vi "getFTData.vi"(4 "Transformed Calibration Matrix":dbl[][](array[numeric]), 5 "error in":errorcluster, 6 "Bias Vector":dbl[](array[numeric])=[0.0, 0.0, 0.0, 0.0, 0.0, 0.0], 7 "Timing parameters":T1={"Sample Rate"=1000.0, "Samples to Read"=100}, 8 "task in":refnum<k21>) -> (0 "error out":errorcluster, 1 "Voltages":dbl[][](array[numeric]), 2 "F/T":dbl[][](array[numeric]) format="%0.4f", 3 "task out 2":refnum<k21>)   [LabVIEW 2012]
uses:
  <vilib>/DAQmx/read.llb/DAQmx Read (Analog 2D DBL NChan NSamp).vi
  <vilib>/DAQmx/miscellaneous.llb/DAQmx Fill In Error Info.vi
  <vilib>/Analysis/baseanly.llb/A x Vector.vi
  <vilib>/Analysis/NI_AALBase.lvlib
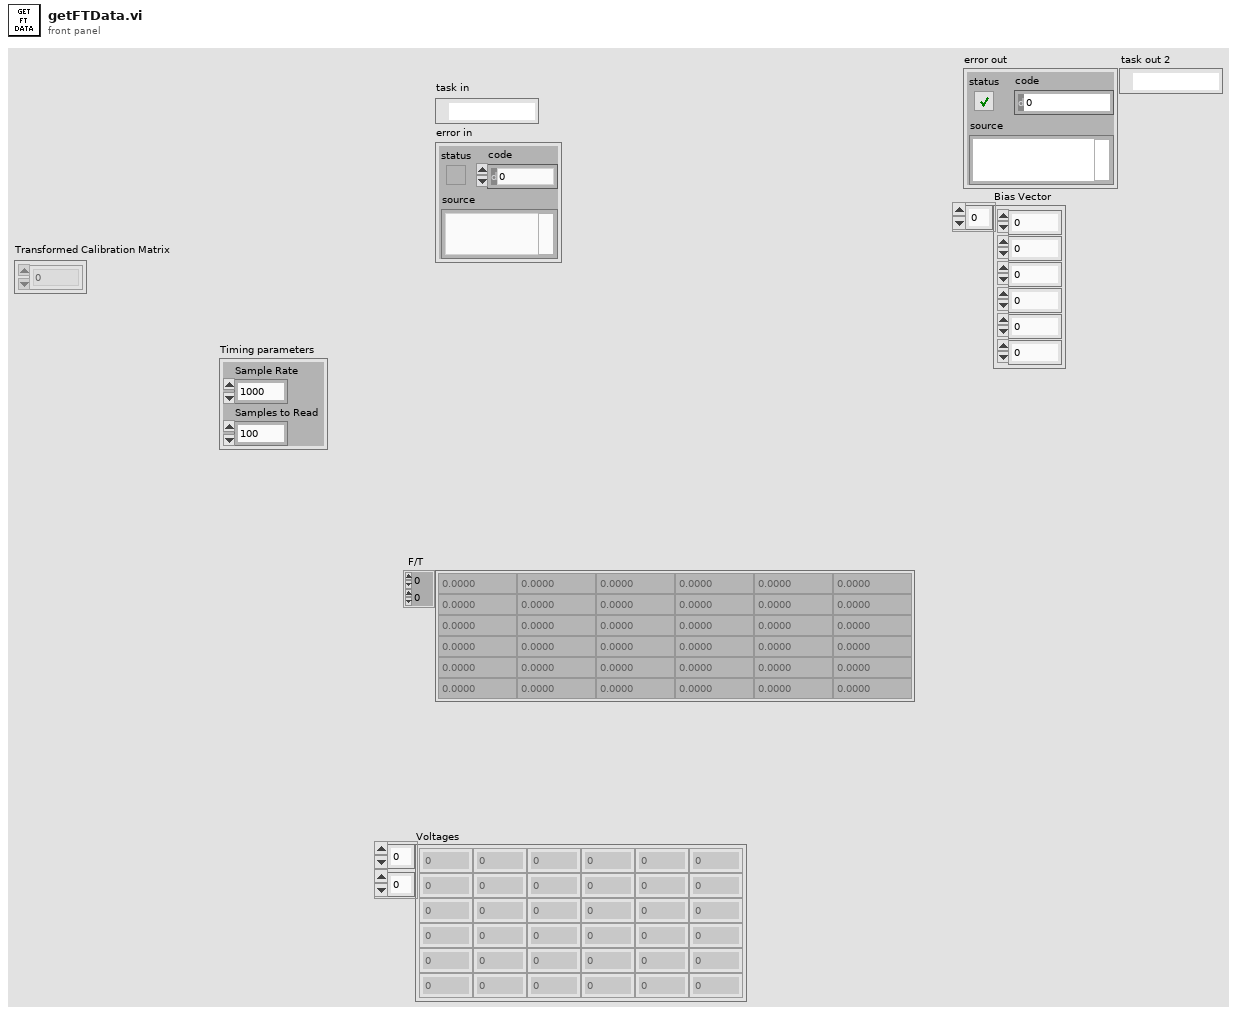
[diagram p1: front panel]
types:
  T1 = cluster{"Sample Rate":dbl, "Samples to Read":i32}
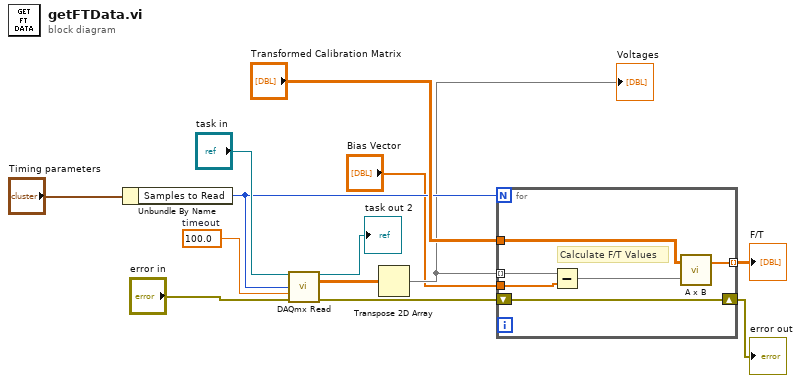
[diagram p0: block diagram]
diagram:
  w6 = 100.0  # timeout
  n1 = Unbundle By Name("Timing parameters") -> ("Samples to Read"=w9:i32)
  n2 = call-poly <vilib>:"DAQmx Read.vi"("task/channels in"="task in", "number of samples per channel"=w9, "timeout"=w6, "error in"="error in") -> ("task out"=→"task out 2":refnum<k21>, "data"=w4:dbl[][], "error out"=w5:errorcluster)  [unwired: 9 in]
  n3 = Transpose 2D Array(2D array=w4) -> (transposed array=w2:dbl[][])
  "Voltages" <- w2
  n4 = for {
    N: w9 -> [_]
    tunnel: [w17] -> w3 mode=indexing
    shift-right: [w16] -> w7
    shift-left: w5 -> [w16]
    tunnel: w2 -> [w19] mode=indexing
    tunnel: "Transformed Calibration Matrix" -> [w15]
    tunnel: "Bias Vector" -> [w14]
    # "Calculate F/T Values"
    n5 = Subtract(x=w19, y=w14) -> (x-y=w18:dbl[])
    n6 = call-poly <vilib>:"A x B.vi"("Vector"=w18, "A"=w15) -> ("A x Vector"=w17:dbl[])  [unwired: 1 out]
  }
  "error out" <- w7
  "F/T" <- w3
